vi "betterRecursiveParse.vi"(10 "XML String in":string, 11 "Control in":refnum<vi>) -> ()   [LabVIEW 2015]
uses:
  <vilib>/NI/GXML/_subVIs/GXML SearchParser/Search Parser.vi
  <vilib>/Utility/Data Type/NI_Data Type.lvlib
  <vilib>/NI/GXML/GXML.lvlib
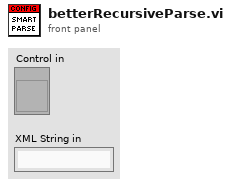
[diagram p1: front panel]
types:
  T1 = typedef "NI_Data Type.lvlib/Data Type.ctl" = enum8{"Invalid Type", "Void", "I8", "I16", "I32", "I64", "U8", "U16", "U32", "U64", "Single Float", "Double Float", "Extended Float", "Single Complex", "Double Complex", "Extended Complex", "Enum U8", "Enum U16", "Enum U32", "Enum U64", "Single Float With Unit", "Double Float With Unit", "Extended Float With Unit", "Single Complex with Unit", "Double Complex with Unit", "Extended Complex with Unit", "Boolean", "String", "Path", "Picture", "Tag", "Array", "Cluster", "Variant", "LV Variant", "Waveform", "Timestamp", "Digital Waveform", "Digital Data", "ExpressData", "Refnum", "External Data", "VI", "Poly VI", "LabVIEW Class Instance", "Fixed Point"}
  T2 = typedef "GXML.lvlib/Item Data.ctl" = cluster{"Item 'Name'":string, "Item Attributes":string, "Item Contents":string}
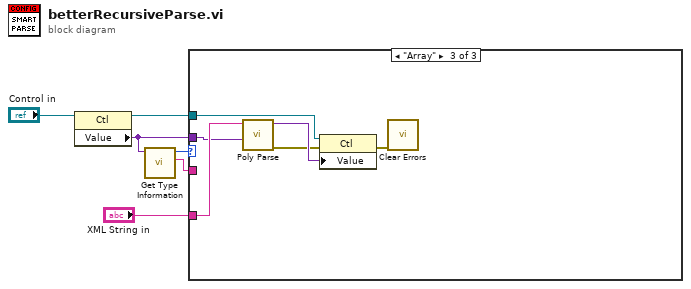
[diagram p0: block diagram]
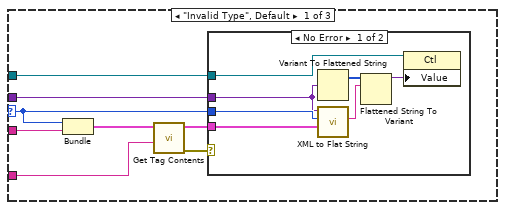
[diagram p2: hidden frame]
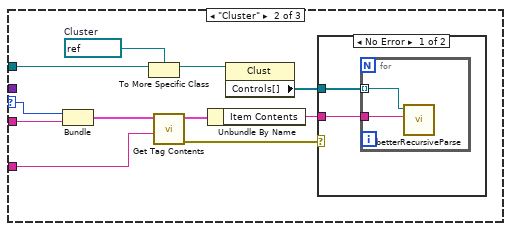
[diagram p4: hidden frame]
diagram:
  n1 = property class="Ctl"(reference="Control in") -> (reference out=w2:refnum<vi>, "Value"=w1:variant)  [unwired: 1 in, 1 out]
  n2 = call <vilib>:"Get Type Information.vi"("Variant"=w1) -> ("Name"=w3:string, "Type"=w5:T1)  [unwired: 6 in, 3 out]
  n3 = case shown="\"Array\"" w5 {
    selector: w5 -> [w11 w31 _]
    tunnel: "XML String in" -> [w10 w28 w42]
    tunnel: w3 -> [w13 w32 _]
    tunnel: w2 -> [w8 w27 w40]
    tunnel: w1 -> [w9 _ w41]
    frame "Invalid Type", Default {
      n4 = Bundle("Type"=w11, "Name"=w13) -> (w14:cluster{"Type":T1, "Name":string})  [unwired: 1 in]
      n5 = call <vilib>:"Get Tag Contents.vi"("Item XML"=w10, "Item Name/Type"=w14) -> ("error out"=w7:errorcluster, "Item XML Data"=w12:T2)  [unwired: 7 in, 1 out]
      n6 = case shown="No Error" w7 {
        tunnel: w12 -> [w21 _]
        tunnel: w11 -> [w20 _]
        tunnel: w9 -> [w19 _]
        tunnel: w8 -> [w16 _]
        frame No Error {
          n7 = Variant To Flattened String(Variant=w19) -> (1:w18:i16[])  [unwired: 1 out]
          n8 = call <vilib>:"XML to Flat String.vi"("Item XML Data"=w21, "Type Enum"=w20, "Item Type Desc"=w19) -> ("XML Data (Flat Str)"=w17:string)  [unwired: 7 in, 1 out]
          n9 = Flattened String To Variant(6:w17, 7:w18) -> (3:w15:variant)  [unwired: 1 in, 1 out]
          n10 = property class="Ctl"(reference=w16, "Value"=w15) -> ()  [unwired: 1 in, 2 out]
        }
        frame Error {
        }
      }
    }
    frame "Cluster" {
      w26 = refnum<vi> refnum  # Cluster
      n11 = Bundle("Type"=w31, "Name"=w32) -> (w30:cluster{"Type":T1, "Name":string})  [unwired: 1 in]
      n12 = To More Specific Class(target class=w26, reference=w27) -> (specific class reference=w23:refnum<vi>)  [unwired: 1 in, 1 out]
      n13 = call <vilib>:"Get Tag Contents.vi"("Item XML"=w28, "Item Name/Type"=w30) -> ("error out"=w25:errorcluster, "Item XML Data"=w29:T2)  [unwired: 7 in, 1 out]
      n14 = Unbundle By Name(w29) -> ("Item Contents"=w24:string)
      n15 = property class="Clust"(reference=w23) -> ("Controls[]"=w22:refnum<vi>[])  [unwired: 1 in, 2 out]
      n16 = case shown="No Error" w25 {
        tunnel: w24 -> [w34 _]
        tunnel: w22 -> [w33 _]
        frame No Error {
          n17 = for {
            tunnel: w34 -> [w36]
            tunnel: w33 -> [w35] mode=indexing
            n18 = call "betterRecursiveParse.vi"("XML String in"=w36, "Control in"=w35) -> ()  [unwired: 10 in]
          }
        }
        frame Error {
        }
      }
    }
    frame "Array" {
      n19 = call-poly <vilib>:"Poly Parse.vi"("TypeDesc"=w41, "XML String In"=w42) -> ("error out"=w38:errorcluster, "Parsed Data"=w39:variant)  [unwired: 8 in]
      n20 = property class="Ctl"(reference=w40, error in=w38, "Value"=w39) -> (error out=w37:errorcluster)  [unwired: 1 out]
      n21 = call <vilib>:"Clear Errors.vi"("error in (no error)"=w37) -> ()  [unwired: 5 in, 2 out]
    }
  }
